vi "getState.vi"(8 "error in (no error)":errorcluster, 11 "Model in":refnum<class "Model.lvclass">) -> (0 "error out":errorcluster, 2 "State out":refnum<class "State.lvclass">, 3 "Model out":refnum<class "Model.lvclass">)   [LabVIEW 2016, in "Model.lvclass"]
uses:
  Model.lvclass
  States/State/State.lvclass
  Model.lvclass/Model.ctl
  States/StateFactory/StateFactory.lvclass/StateFactory.ctl
  States/OfflineState/OfflineState.lvclass
  D:/Code/ts_M1M3Support/States/State/State.lvclass
  States/InitialState/InitialState.lvclass
  States/StandbyState/StandbyState.lvclass
  States/DisabledState/DisabledState.lvclass
  States/ParkedState/ParkedState.lvclass
  States/FaultState/FaultState.lvclass
  States/ParkedMaintenanceState/ParkedMaintenanceState.lvclass
  States/ActiveMaintenanceState/ActiveMaintenanceState.lvclass
  States/StateFactory/StateFactory.lvclass
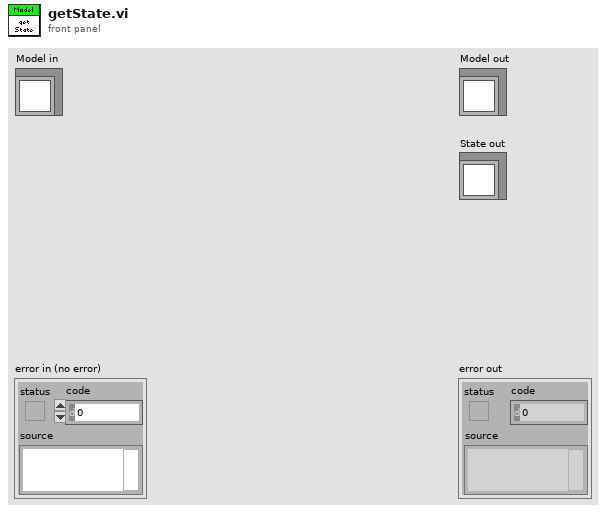
[diagram p1: front panel]
types:
  T1 = typedef "M1M3SupportTopics.lvlib/DetailedStates.ctl" = enum16{"OfflineState", "InitialState", "StandbyState", "DisabledState", "ParkedState", "FaultState", "ParkedMaintenanceState", "ActiveMaintenanceState"}
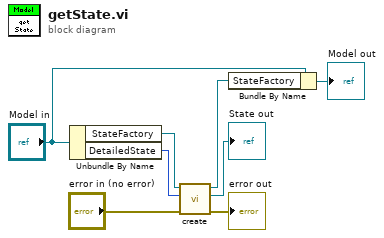
[diagram p0: block diagram]
diagram:
  n1 = Unbundle By Name("Model in") -> ("StateFactory"=w6:refnum<class "StateFactory.lvclass">, "DetailedState"=w7:T1)
  n2 = call "create.vi"("error in (no error)"="error in (no error)", "DetailedStates"=w7, "StateFactory in"=w6) -> ("error out"=→"error out":errorcluster, "State out"=→"State out":refnum<class "State.lvclass">, "StateFactory out"=w5:refnum<class "StateFactory.lvclass">)  [unwired: 6 in]
  n3 = Bundle By Name(cluster="Model in", "StateFactory"=w5) -> (→"Model out":refnum<class "Model.lvclass">)
